vi "server_pos_indicator.vi"(5 "reset":bool, 6 "tentative":bool, 7 "rough":bool, 8 "error in":errorcluster, 10 "yc":dbl format="%#_6p", 11 "xc":dbl format="%#_6p") -> (0 "error out":errorcluster)   [LabVIEW 2014]
uses:
  <vilib>/Utility/file.llb/Write To Spreadsheet File (DBL).vi
panel:
  out "rough Array":bool[](array[boolean])
  out "num_rough":i32
  out "size(s)":i32
  out "output array":T1(array[cluster])
  out "position":picture
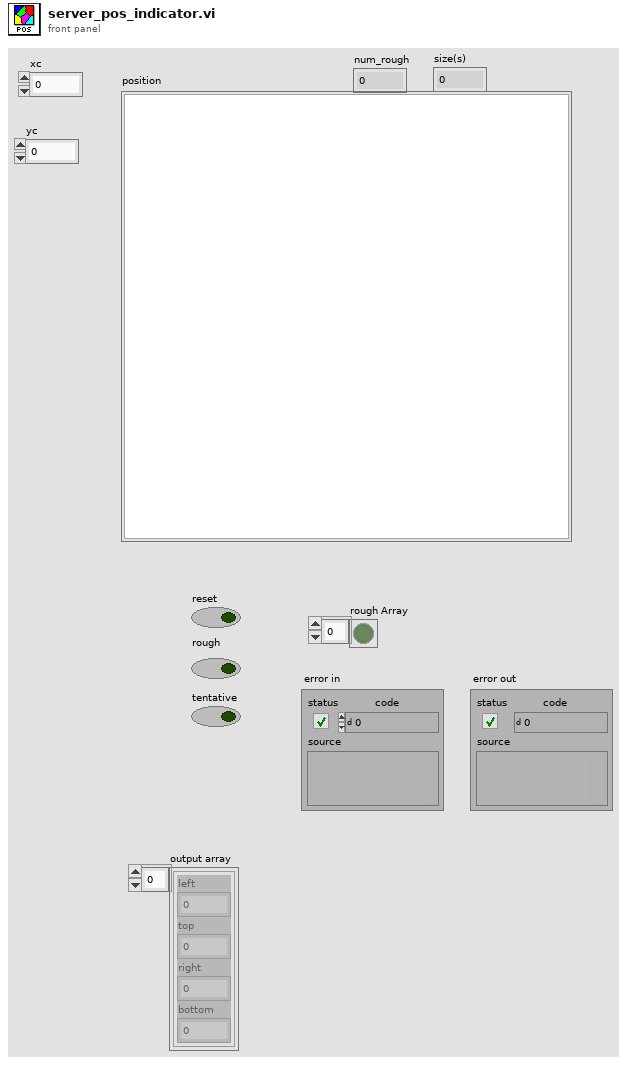
[diagram p1: front panel]
types:
  T1 = cluster{"left":i16, "top":i16, "right":i16, "bottom":i16}[]
  T2 = cluster{"horizontal":enum16{"left", "center", "right"}, "vertical":enum16{"top", "center", "bottom"}}
  T3 = cluster{"left":i16, "top":i16, "right":i16, "bottom":i16}
  T4 = cluster{"Width":u16, "Style":enum32{"Solid", "Dash", "Dot", "DashDot", "DashDotDot"}}
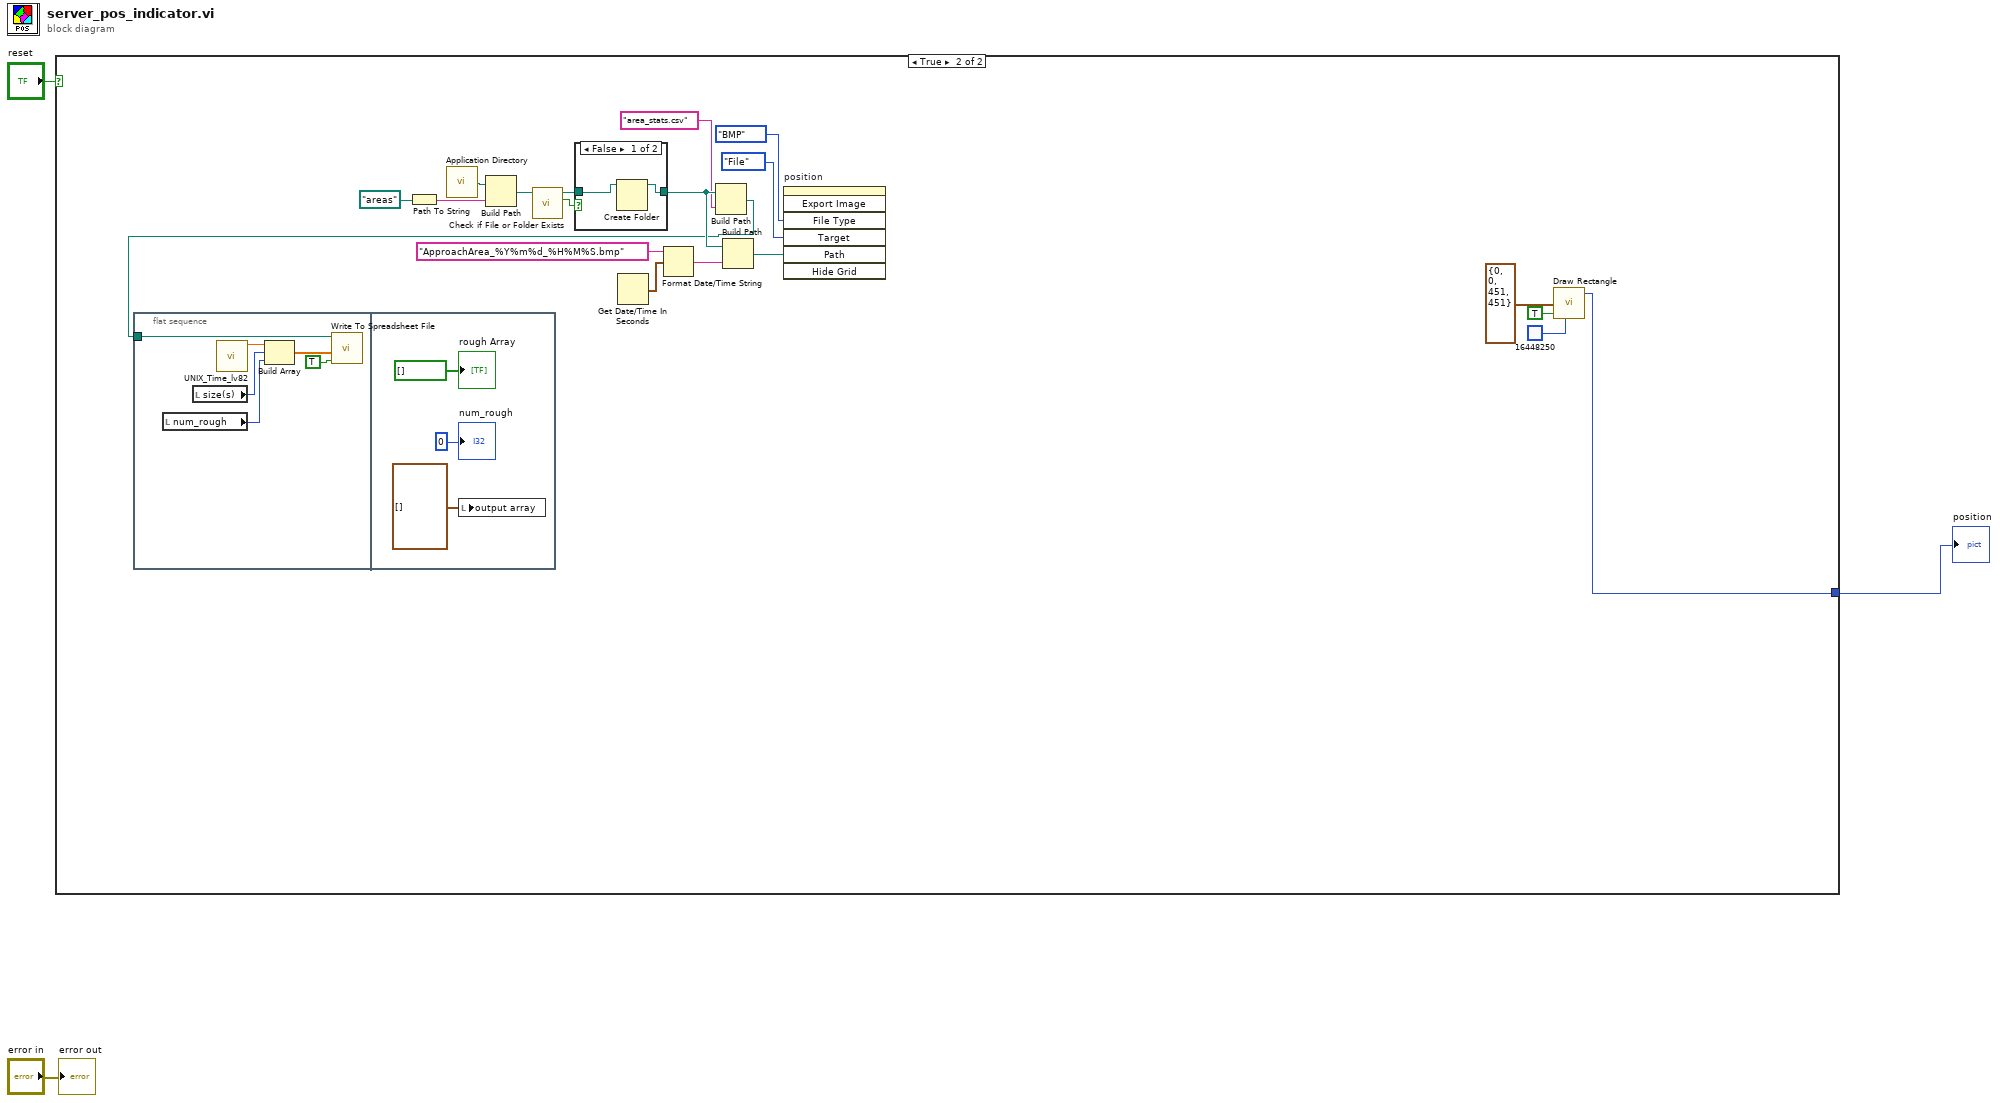
[diagram p0: block diagram]
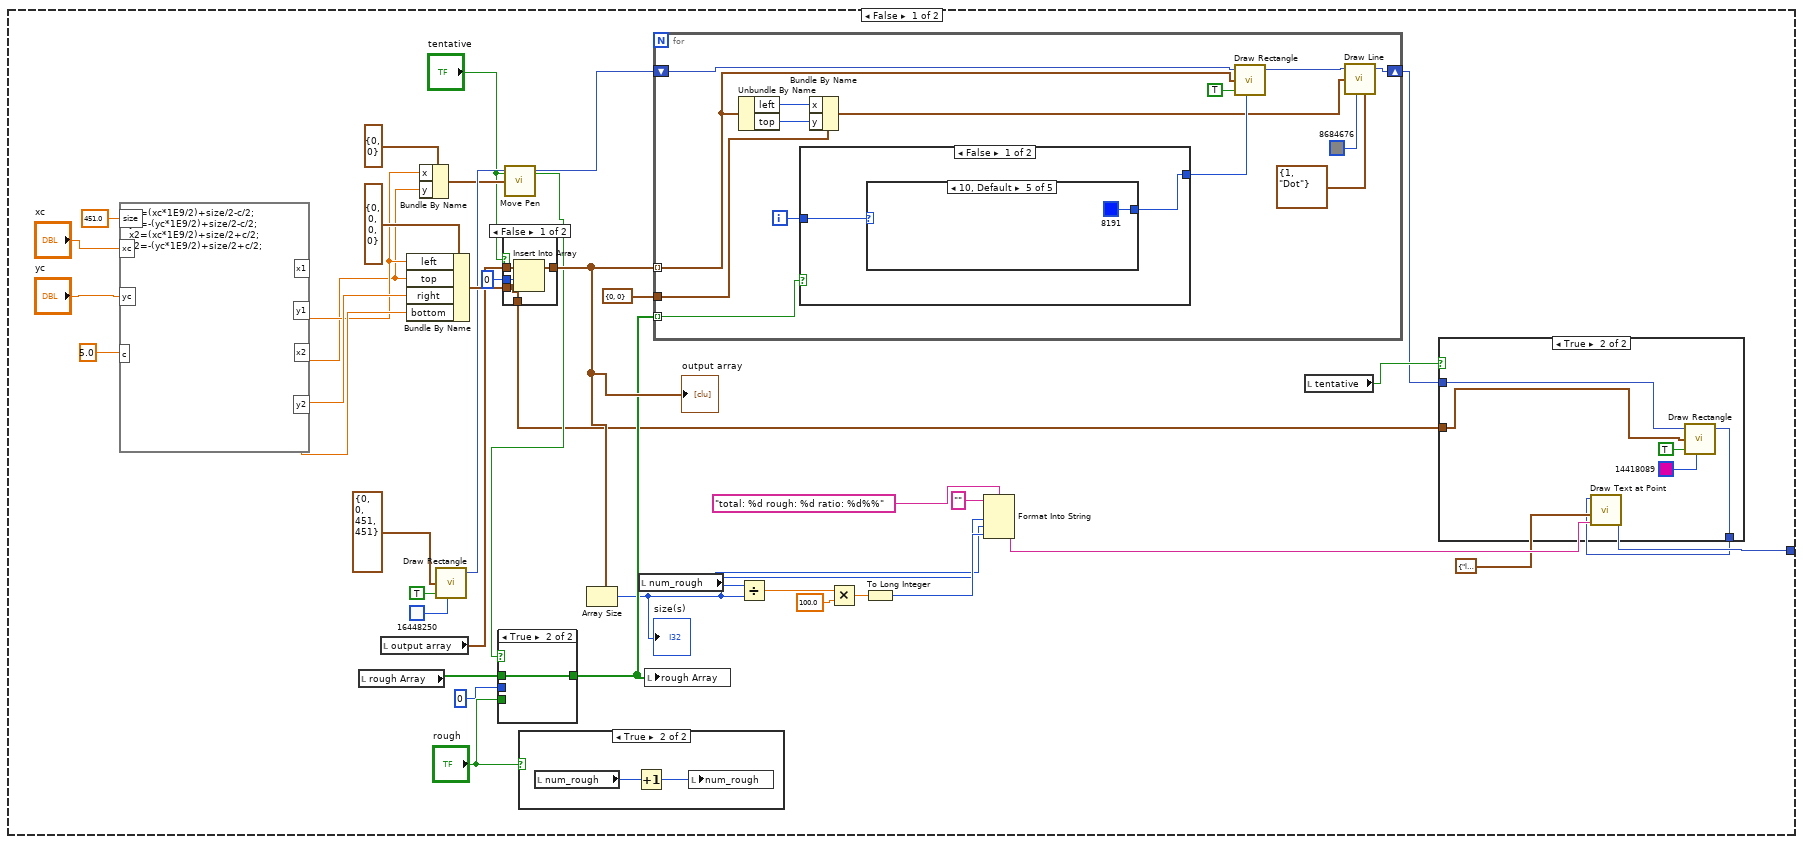
[diagram p2: hidden frame]
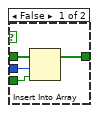
[diagram p4: hidden frame]
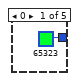
[diagram p7: hidden frame]
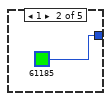
[diagram p8: hidden frame]
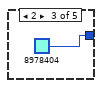
[diagram p9: hidden frame]
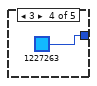
[diagram p10: hidden frame]
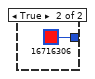
[diagram p11: hidden frame]
diagram:
  n1 = case shown="True" "reset" {
    tunnel: [w20 w101] -> w2
    frame False {
      n2 = formula code="x1=(xc*1E9/2)+size/2-c/2;\ny1=-(yc*1E9/2)+size/2-c/2;\nx2=(xc*1E9/2)+size/2+c/2;\ny2=-(yc*1E9/2)+size/2+c/2;"("xc"="xc", "yc"="yc", "c"=5.0 ("input variable"), "size"=451.0 ("input variable")) -> ("x1"=w12:dbl, "y1"=w11:dbl, "x2"=w40:dbl, "y2"=w39:dbl)
      n3 = local read "rough Array"() -> (w32:bool[])
      n4 = local read "output array"() -> (w33:T1)
      n5 = Bundle By Name(cluster=T3 {"left"=0, "top"=0, "right"=0, "bottom"=0} ("rect"), "left"=w12, "top"=w11, "right"=w40, "bottom"=w39) -> (w35:T3)
      n6 = Bundle By Name(cluster=cluster{"x":i16, "y":i16} {"x"=0, "y"=0} ("end point"), "x"=w12, "y"=w11) -> (w14:cluster{"x":i16, "y":i16})
      n7 = call <vilib>:"Draw Rectangle.vi"("rect"=T3 {"left"=0, "top"=0, "right"=451, "bottom"=451}, "fill?(F)"=TRUE, "color(black)"=u32 16448250) -> ("new picture"=w16:picture)  [unwired: 6 in]
      n8 = case shown="True" "tentative" {
        tunnel: w32 -> [w54 w55]
        tunnel: [w53 w55] -> w31
        tunnel: "rough" -> [w52 _]
        tunnel: 0 ("index") -> [w51 _]
        frame False {
          n9 = Insert Into Array(array=w54, index=w51, new element=w52) -> (w53:bool[])
        }
        frame True {
        }
      }
      n10 = case shown="False" "tentative" {
        tunnel: w35 -> [w56 w60]
        tunnel: [w59 w61] -> w34
        tunnel: w33 -> [w58 w61]
        tunnel: 0 ("index") -> [w57 _]
        tunnel: [w56 w60] -> w5
        frame False {
          n11 = Insert Into Array(array=w58, index=w57, new element=w56) -> (w59:T1)
        }
        frame True {
        }
      }
      "output array" <- w34
      n12 = call <vilib>:"Move Pen.vi"("new position"=w14, "picture"=w16) -> ("new picture"=w15:picture)  [unwired: 3 in]
      n13 = case shown="True" "rough" {
        frame False {
        }
        frame True {
          n14 = local read "num_rough"() -> (w63:i32)
          n15 = Increment(x=w63) -> (x+1=w62:i32)
          n16 = local write "num_rough"(w62) -> ()
        }
      }
      n17 = Array Size(array=w34) -> (size(s)=w19:i32)
      "size(s)" <- w19
      n18 = local read "num_rough"() -> (w21:i32)
      n19 = local write "rough Array"(w31) -> ()
      n20 = for {
        shift-right: [w66] -> w7
        shift-left: w15 -> [w77]
        tunnel: w34 -> [w72] mode=indexing
        tunnel: w31 -> [w73] mode=indexing
        tunnel: cluster{"x":i16, "y":i16} {"x"=0, "y"=0} ("end point") -> [w70]
        i -> [w76]
        n21 = Unbundle By Name(w72) -> ("left"=w69:i16, "top"=w68:i16)
        n22 = case shown="False" w73 {
          tunnel: w76 -> [w79 _]
          tunnel: [w78 u32 16716306 ("color(black)")] -> w74
          frame False {
            n23 = case shown="10, Default" w79 {
              tunnel: [u32 65323 ("color(black)") u32 61185 ("color(black)") u32 8978404 ("color(black)") u32 1227263 ("color(black)") u32 8191 ("color(black)")] -> w78
              frame 0 {
              }
              frame 1 {
              }
              frame 2 {
              }
              frame 3 {
              }
              frame 10, Default {
              }
            }
          }
          frame True {
          }
        }
        n24 = Bundle By Name(cluster=w70, "x"=w69, "y"=w68) -> (w71:cluster{"x":i16, "y":i16})
        n25 = call <vilib>:"Draw Rectangle.vi"("picture"=w77, "rect"=w72, "fill?(F)"=TRUE, "color(black)"=w74) -> ("new picture"=w67:picture)  [unwired: 5 in]
        n26 = call <vilib>:"Draw Line.vi"("picture"=w67, "end point"=w71, "color(black)"=u32 8684676, "pen"=T4 {"Width"=1, "Style"=enum."Dot"}) -> ("new picture"=w66:picture)  [unwired: 5 in]
      }
      n27 = Divide(x=w21, y=w19) -> (x/y=w26:dbl)
      n28 = Multiply(x=w26, y=100.0) -> (x*y=w24:dbl)
      n29 = To Long Integer(number=w24) -> (32bit integer=w23:i32)
      n30 = Format Into String(format string="total: %d rough: %d ratio: %d%%", initial string="", w19, w21, w23) -> (resulting string=w22:string)  [unwired: 1 in, 1 out]
      n31 = local read "tentative"() -> (w8:bool)
      n32 = case shown="True" w8 {
        tunnel: w7 -> [w45 w50]
        tunnel: [w45 w47] -> w6
        tunnel: w5 -> [_ w46]
        frame False {
        }
        frame True {
          n33 = call <vilib>:"Draw Rectangle.vi"("picture"=w50, "rect"=w46, "fill?(F)"=TRUE, "color(black)"=u32 14418089) -> ("new picture"=w47:picture)  [unwired: 5 in]
        }
      }
      n34 = call <vilib>:"Draw Text at Point.vi"("text"=w22, "alignment(left, top)"=T2 {"horizontal"=enum."left", "vertical"=enum."top"}, "picture"=w6) -> ("new picture"=w20:picture)  [unwired: 7 in, 1 out]
    }
    frame True {
      n35 = flat-sequence {
        tunnel: w86 -> [w110]
        frame #0 {
          n36 = local read "num_rough"() -> (w106:i32)
          n37 = local read "size(s)"() -> (w107:i32)
          n38 = call "UNIX_Time_lv82.vi"() -> ("Unix time"=w105:dbl)  [unwired: 10 in, 1 out]
          n39 = Build Array(w105, w107, w106) -> (w108:dbl[])
          n40 = call-poly <vilib>:"Write To Spreadsheet File.vi"("append to file? (new file:F)"=TRUE, "1D data"=w108, "file path (dialog if empty)"=w110) -> ()  [unwired: 5 in, 1 out]
        }
        frame #1 {
          n41 = local write "output array"(T1 [] ("output array")) -> ()
          "num_rough" <- 0 ("rough")
          "rough Array" <- bool[] []
        }
      }
      n42 = Path To String(path=path "areas") -> (string=w93:string)
      n43 = call <vilib>:"Application Directory.vi"() -> ("Application Directory"=w95:path)
      n44 = Build Path(base path=w95, name or relative path=w93) -> (appended path=w90:path)
      n45 = call <vilib>:"Check if File or Folder Exists.vi"("path"=w90) -> ("file or folder exists?"=w91:bool, "dup path"=w92:path)  [unwired: 8 in, 1 out]
      n46 = case shown="False" w91 {
        tunnel: w92 -> [w115 w116]
        tunnel: [w114 w116] -> w88
        frame False {
          n47 = Create Folder(path (use dialog)=w115) -> (created path=w114:path)  [unwired: 2 in, 2 out]
        }
        frame True {
        }
      }
      n48 = Get Date/Time In Seconds() -> (seconds since 1Jan1904=w89:timestamp)
      n49 = Format Date/Time String(time format string (%c)="ApproachArea_%Y%m%d_%H%M%S.bmp", seconds (now)=w89) -> (date/time string=w99:string)  [unwired: 1 in]
      n50 = Build Path(base path=w88, name or relative path="area_stats.csv") -> (appended path=w86:path)
      n51 = Build Path(base path=w88, name or relative path=w99) -> (appended path=w96:path)
      n52 = invoke on="position" class="Pict" method="Export Image"("File Type"=enum32{"BMP", "EPS", "EMF", "PICT"}."BMP", "Target"=enum32{"File", "Clipboard"}."File", "Path"=w96) -> ()  [unwired: 4 in, 7 out]
      n53 = call <vilib>:"Draw Rectangle.vi"("rect"=T3 {"left"=0, "top"=0, "right"=451, "bottom"=451}, "fill?(F)"=TRUE, "color(black)"=u32 16448250) -> ("new picture"=w101:picture)  [unwired: 6 in]
    }
  }
  "position" <- w2
  "error out" <- "error in"
